vi "PointROIToLineROI.vi"(6 "Scan Settings":T3, 8 "Number of Lines (Odd)":i32, 9 "Line Length (pixels)":i32, 10 "Line Offset X (pixels)":i32, 11 "PT ROIs":T1(array[cluster])) -> (3 "LINE ROIs":T1(array[cluster]))   [LabVIEW 2014]
panel:
  in  "Cluster":T2
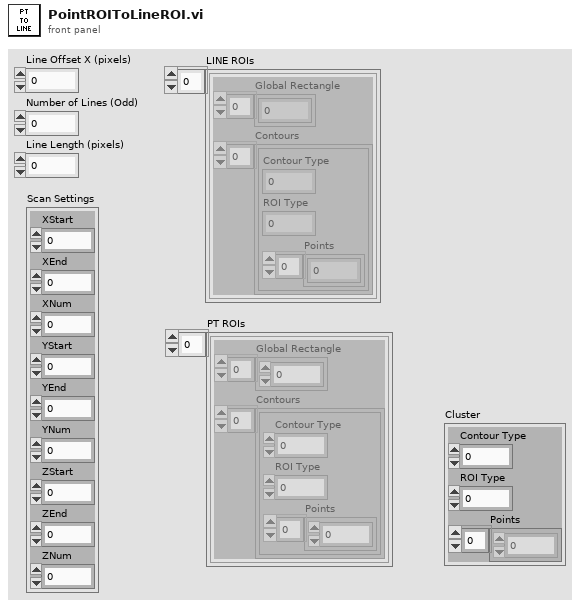
[diagram p1: front panel]
types:
  T1 = cluster{"Global Rectangle":i32[], "Contours":cluster{"Contour Type":u32, "ROI Type":u32, "Points":i32[]}[]}[]
  T2 = cluster{"Contour Type":u32, "ROI Type":u32, "Points":i32[]}
  T3 = cluster{"XStart":i32, "XEnd":i32, "XNum":i32, "YStart":i32, "YEnd":i32, "YNum":i32, "ZStart":i32, "ZEnd":i32, "ZNum":i32}
  T4 = cluster{"Global Rectangle":i32[], "Contours":cluster{"Contour Type":u32, "ROI Type":u32, "Points":i32[]}[]}
  T5 = cluster{"Contour Type":u32, "ROI Type":u32, "Points":i32[]}[]
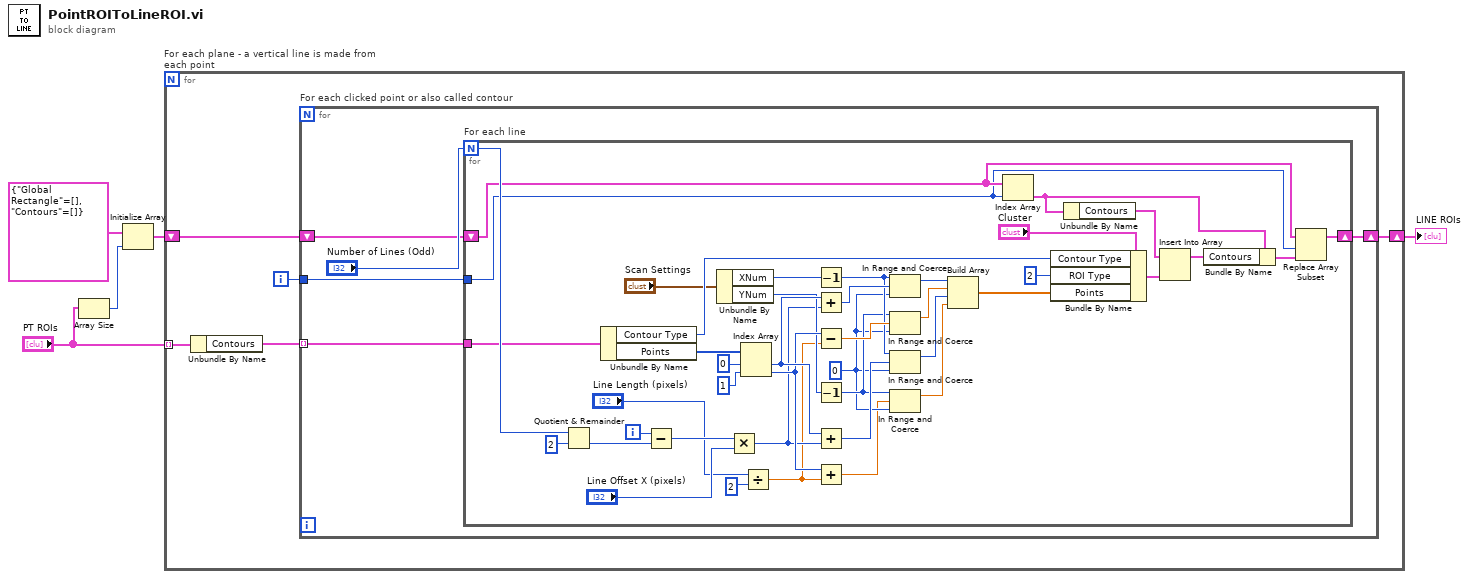
[diagram p0: block diagram]
diagram:
  n1 = Array Size(array="PT ROIs") -> (size(s)=w2:i32)
  n2 = Initialize Array(T4 {"Global Rectangle"=[], "Contours"=[]} ("ROI"), w2) -> (w4:T1)
  n3 = for "For each plane - a vertical line is made from each point" {
    shift-right: [w7] -> w1
    shift-left: w4 -> [w9]
    tunnel: "PT ROIs" -> [w10] mode=indexing
    i -> [w6]
    n4 = Unbundle By Name(w10) -> ("Contours"=w8:T5)
    n5 = for "For each clicked point or also called contour" {
      tunnel: w8 -> [w14] mode=indexing
      shift-right: [w12] -> w7
      shift-left: w9 -> [w13]
      tunnel: w6 -> [w11]
      n6 = for "For each line" {
        N: "Number of Lines (Odd)" -> [w51]
        tunnel: w14 -> [w47]
        shift-right: [w32] -> w12
        shift-left: w13 -> [w34]
        tunnel: w11 -> [w31]
        i -> [w52]
        w18 = 0 ("y")
        n7 = Quotient & Remainder(x=w51, y=2) -> (floor(x/y)=w53:i32)  [unwired: 1 out]
        n8 = Unbundle By Name(w47) -> ("Contour Type"=w44:u32, "Points"=w45:i32[])
        n9 = Subtract(x=w52, y=w53) -> (x-y=w48:i32)
        n10 = Unbundle By Name("Scan Settings") -> ("XNum"=w40:i32, "YNum"=w39:i32)
        n11 = Multiply(x=w48, y="Line Offset X (pixels)") -> (x*y=w30:i32)
        n12 = Index Array(array=w45, index #1=0 ("index"), index #2=1 ("index")) -> (element #1=w55:i32, element #2=w54:i32)
        n13 = Divide(x="Line Length (pixels)", y=2) -> (x/y=w29:dbl)
        n14 = Decrement(x=w40) -> (x-1=w22:i32)
        n15 = Add(x=w55, y=w30) -> (x+y=w26:i32)
        n16 = Subtract(x=w54, y=w29) -> (x-y=w24:dbl)
        n17 = Decrement(x=w39) -> (x-1=w19:i32)
        n18 = Add(x=w55, y=w30) -> (x+y=w21:i32)
        n19 = Add(x=w54, y=w29) -> (x+y=w17:dbl)
        n20 = In Range and Coerce(upper limit=w22, x=w26, lower limit=w18) -> (coerced(x)=w25:i32)  [unwired: 1 out]
        n21 = In Range and Coerce(upper limit=w19, x=w24, lower limit=w18) -> (coerced(x)=w23:dbl)  [unwired: 1 out]
        n22 = In Range and Coerce(upper limit=w22, x=w21, lower limit=w18) -> (coerced(x)=w20:i32)  [unwired: 1 out]
        n23 = In Range and Coerce(upper limit=w19, x=w17, lower limit=w18) -> (coerced(x)=w16:dbl)  [unwired: 1 out]
        n24 = Build Array(w25, w23, w20, w16) -> (w42:dbl[])
        n25 = Index Array(array=w34, index=w31) -> (element=w36:T4)
        n26 = Bundle By Name(cluster="Cluster", "Contour Type"=w44, "ROI Type"=u32 2, "Points"=w42) -> (w38:T2)
        n27 = Unbundle By Name(w36) -> ("Contours"=w37:T5)
        n28 = Insert Into Array(array=w37, new element=w38) -> (w35:T5)  [unwired: 1 in]
        n29 = Bundle By Name(cluster=w36, "Contours"=w35) -> (w33:T4)
        n30 = Replace Array Subset(array=w34, new element=w33, index=w31) -> (w32:T1)
      }
    }
  }
  "LINE ROIs" <- w1
